vi "Delay_second.vi"(1 "Delay":dbl, 3 "error in (no error)":errorcluster) -> (10 "error out":errorcluster)   [LabVIEW 8.6]
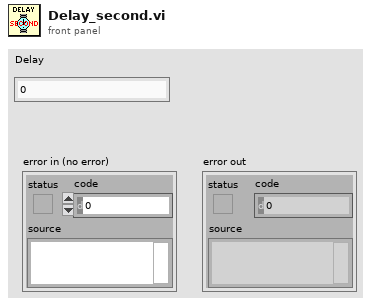
[diagram p1: front panel]
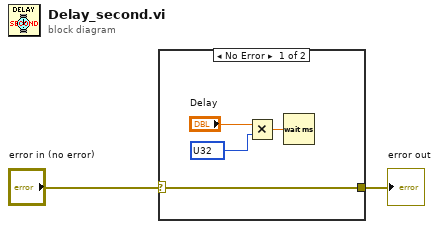
[diagram p0: block diagram]
diagram:
  n1 = case shown="No Error" "error in (no error)" {
    selector: "error in (no error)" -> [w6 w7]
    tunnel: [w6 w7] -> w1
    frame #0 {
      n2 = Multiply(x="Delay", y=u32 ?) -> (x*y=w5:dbl)
      n3 = Wait (ms)(milliseconds to wait=w5) -> ()  [unwired: 1 out]
    }
    frame #1 {
    }
  }
  "error out" <- w1
